vi "Query Multi Eval Meas List TPower Limit Check Results.vi"(8 "error in (no error)":errorcluster, 9 "Result Type (Current)":i32(ring) items=["Current"=0, "Average"=1, "Maximum"=4, "Minimum"=5], 10 "Instance (1)":T1=1, 11 "VISA resource name":refnum<visa-resource-name>) -> (0 "error out":errorcluster, 1 "TPower Limit Check Results":i32[](array[numeric]), 2 "Reliability":i32, 3 "VISA resource name out":refnum<visa-resource-name>)   [LabVIEW 2015, in "Rohde&Schwarz CMXP NR FR2 Measurement.lvlib"]
doc: "Returns the limit check results for the user equipment power values for all measured list mode segments.\n\nAttributes:\nRSCMXPNRFR2M_ATTR_QUERY_MULTI_EVAL_MEASUREMENT_LIST_TPOWER_AVERAGE_LIMIT_CHECK_RESULTS\nRSCMXPNRFR2M_ATTR_QUERY_MULTI_EVAL_MEASUREMENT_LIST_TPOWER_CURRENT_LIMIT_CHECK_RESULTS\nRSCMXPNRFR2M_ATTR_QUERY_MULTI_EVAL_MEASUREMENT_LIST_TPOWER_MAXIMUM_LIMIT_CHECK_RESULTS\nRSCMXPNRFR2M_ATTR_QUERY_MULTI_EVAL_MEASUREMENT_LIST_TPOWER_MINIMUM_LIMIT_CHECK_RESULTS\n\nRemote-control commands:\nCALCulate:NRMMw:MEAS<i>:MEValuation:LIST:MODulation:TPOWer:AVERage?\nCALCulate:NRMMw:MEAS<i>:MEValuation:LIST:MODulation:TPOWer:CURRent?\nCALCulate:NRMMw:MEAS<i>:MEValuation:LIST:MODulation:TPOWer:MAXimum?\nCALCulate:NRMMw:MEAS<i>:MEValuation:LIST:MODulation:TPOWer:MINimum?"
uses:
  <instrlib>/Rohde&Schwarz CMXP NR FR2 Measurement/Rohde&Schwarz CMXP NR FR2 Measurement.lvlib
  <instrlib>/Rohde&Schwarz CMXP NR FR2 Measurement/Private/_Instance.ctl
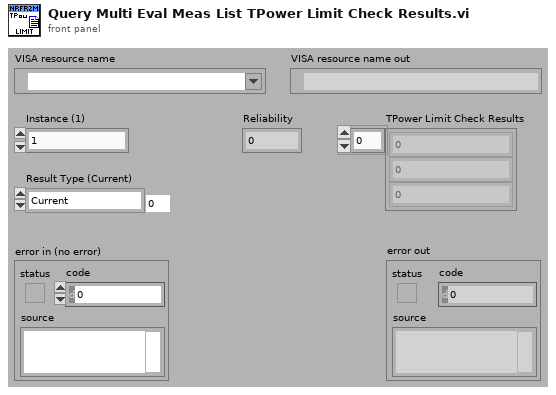
[diagram p1: front panel]
types:
  T1 = typedef "Rohde&Schwarz CMXP NR FR2 Measurement.lvlib/_Instance.ctl" = i32
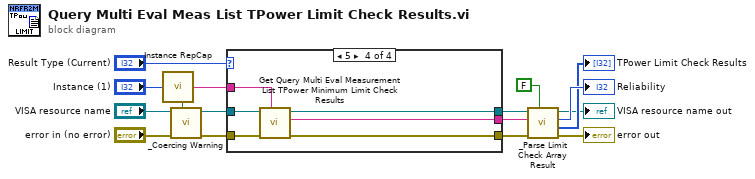
[diagram p0: block diagram]
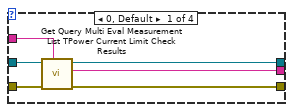
[diagram p2: hidden frame]
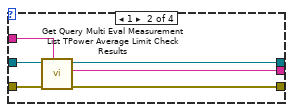
[diagram p3: hidden frame]
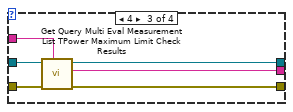
[diagram p4: hidden frame]
diagram:
  n1 = call <instrlib>:"Instance RepCap.vi"("Instance In"="Instance (1)") -> ("In Range?"=w14:bool, "RepCap Identifier Out"=w11:string)  [unwired: 1 in]
  n2 = call <instrlib>:"_Coercing Warning.vi"("In Range?"=w14, "error in (no error)"="error in (no error)", "VISA resource name"="VISA resource name") -> ("error out"=w13:errorcluster, "VISA resource name out"=w12:refnum<visa-resource-name>)  [unwired: 7 in]
  n3 = case shown="5" "Result Type (Current)" {
    tunnel: w13 -> [w22 w28 w34 w40]
    tunnel: w12 -> [w21 w27 w33 w39]
    tunnel: w11 -> [w20 w26 w32 w38]
    tunnel: [w19 w25 w31 w37] -> w9
    tunnel: [w18 w24 w30 w36] -> w8
    tunnel: [w17 w23 w29 w35] -> w7
    frame 0, Default {
      n4 = call "Get Query Multi Eval Measurement List TPower Current Limit Check Results"("Repeated Capabilities"=w20, "error in (no error)"=w22, "instrument handle"=w21) -> ("error out"=w19:errorcluster, "Query Multi Eval Measurement List TPower Current Limit Check Results"=w18:string, "instrument handle out"=w17:refnum<visa-resource-name>)  [unwired: 6 in]
    }
    frame 1 {
      n5 = call "Get Query Multi Eval Measurement List TPower Average Limit Check Results"("Repeated Capabilities"=w26, "error in (no error)"=w28, "instrument handle"=w27) -> ("error out"=w25:errorcluster, "Query Multi Eval Measurement List TPower Average Limit Check Results"=w24:string, "instrument handle out"=w23:refnum<visa-resource-name>)  [unwired: 6 in]
    }
    frame 4 {
      n6 = call "Get Query Multi Eval Measurement List TPower Maximum Limit Check Results"("Repeated Capabilities"=w32, "error in (no error)"=w34, "instrument handle"=w33) -> ("error out"=w31:errorcluster, "Query Multi Eval Measurement List TPower Maximum Limit Check Results"=w30:string, "instrument handle out"=w29:refnum<visa-resource-name>)  [unwired: 6 in]
    }
    frame 5 {
      n7 = call "Get Query Multi Eval Measurement List TPower Minimum Limit Check Results"("Repeated Capabilities"=w38, "error in (no error)"=w40, "instrument handle"=w39) -> ("error out"=w37:errorcluster, "Query Multi Eval Measurement List TPower Minimum Limit Check Results"=w36:string, "instrument handle out"=w35:refnum<visa-resource-name>)  [unwired: 6 in]
    }
  }
  n8 = call <instrlib>:"_Parse Limit Check Array Result.vi"("error in (no error)"=w9, "Input String"=w8, "VISA resource name"=w7, "Out of tolerance? (F)"=FALSE) -> ("error out"=→"error out":errorcluster, "Results"=→"TPower Limit Check Results":i32[], "Reliability"=→"Reliability":i32, "VISA resource name out"=→"VISA resource name out":refnum<visa-resource-name>)  [unwired: 3 in]
